vi "Toolkit - Cluster Constant.vi"() -> ()   [LabVIEW 2017]
doc: "Alphabetizes a cluster constant using VI scripting and the ACE toolkit VIs"
uses:
  <vilib>/Utility/traverseref.llb/TRef TravTarget.ctl
  Toolkit/Toolkit.lvlib
  <vilib>/Utility/traverseref.llb/VI Scripting - Traverse.lvlib
panel:
  out "Change?":bool
  # "Overview: Demonstrates alphabetizing a cluster constant using VI scripting the ACE toolkit\nInstructions:\n1. Run this VI"
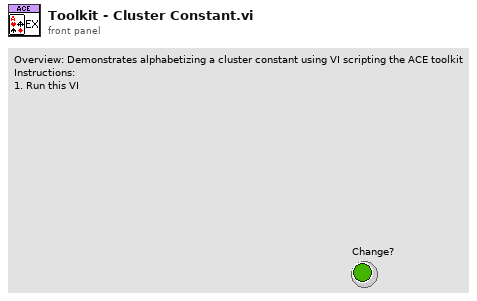
[diagram p1: front panel]
types:
  T1 = enum32{"Invalid", "Standard", "Closed", "Hidden", "Minimized", "Maximized"}
  T2 = typedef "TRef TravTarget.ctl" = enum16{"FP", "BD", "Other"}
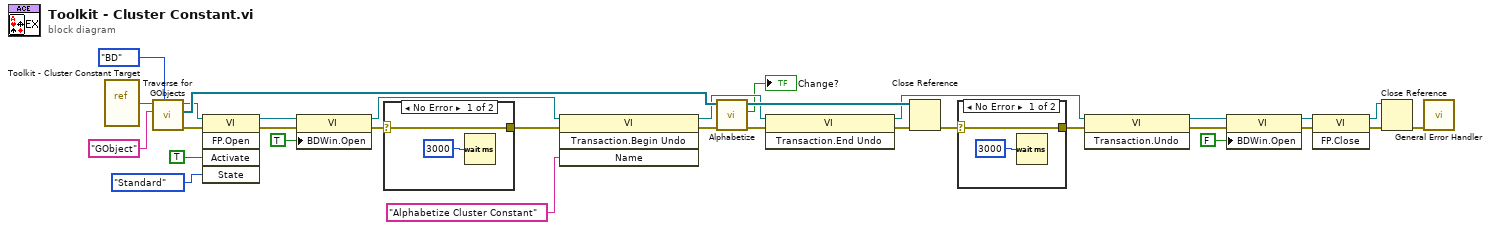
[diagram p0: block diagram]
diagram:
  n1 = vi-ref "Toolkit - Cluster Constant Target.vi"() -> (w17:refnum<vi>)
  n2 = call <vilib>:"Traverse for GObjects.vi"("Traverse Target"=TRef_TravTarget."BD", "Class Name"="GObject", "VI Refnum"=w17) -> ("error out"=w25:errorcluster, "References"=w30:refnum<vi>[], "dup VI Refnum"=w24:refnum<vi>)  [unwired: 5 in, 1 out]
  n3 = invoke class="VI" method="FP.Open"(reference=w24, error in=w25, "Activate"=TRUE ("Activate?"), "State"=T1."Standard") -> (reference out=w23:refnum<vi>, error out=w22:errorcluster)  [unwired: 1 in, 3 out]
  n4 = property class="VI"(reference=w23, error in=w22, "BDWin.Open"=TRUE ("Block Diagram Window:Open")) -> (reference out=w14:refnum<vi>, error out=w20:errorcluster)
  n5 = case shown="No Error" w20 {
    selector: w20 -> [w34 w35]
    tunnel: [w34 w35] -> w16
    frame No Error {
      n6 = Wait (ms)(milliseconds to wait=u32 3000) -> ()  [unwired: 1 out]
    }
    frame Error {
    }
  }
  n7 = invoke class="VI" method="Transaction.Begin Undo"(reference=w14, error in=w16, "Name"="Alphabetize Cluster Constant") -> (reference out=w11:refnum<vi>, error out=w15:errorcluster)  [unwired: 1 in, 2 out]
  n8 = call "Alphabetize.vi"("Error In"=w15, "Clusters In"=w30) -> ("Error Out"=w12:errorcluster, "Change?"=→"Change?":bool, "Clusters Out"=w28:refnum<vi>[])  [unwired: 7 in]
  n9 = invoke class="VI" method="Transaction.End Undo"(reference=w11, error in=w12) -> (reference out=w9:refnum<vi>, error out=w10:errorcluster)  [unwired: 1 in, 1 out]
  n10 = Close Reference(reference=w28, error in (no error)=w10) -> (error out=w19:errorcluster)
  n11 = case shown="No Error" w19 {
    selector: w19 -> [w37 w38]
    tunnel: [w37 w38] -> w18
    frame No Error {
      n12 = Wait (ms)(milliseconds to wait=u32 3000) -> ()  [unwired: 1 out]
    }
    frame Error {
    }
  }
  n13 = invoke class="VI" method="Transaction.Undo"(reference=w9, error in=w18) -> (reference out=w8:refnum<vi>, error out=w7:errorcluster)  [unwired: 1 in, 1 out]
  n14 = property class="VI"(reference=w8, error in=w7, "BDWin.Open"=FALSE ("Block Diagram Window:Open")) -> (reference out=w5:refnum<vi>, error out=w2:errorcluster)
  n15 = invoke class="VI" method="FP.Close"(reference=w5, error in=w2) -> (reference out=w4:refnum<vi>, error out=w3:errorcluster)  [unwired: 1 in, 1 out]
  n16 = Close Reference(reference=w4, error in (no error)=w3) -> (error out=w29:errorcluster)
  n17 = call <vilib>:"General Error Handler.vi"("error in (no error)"=w29) -> ()  [unwired: 10 in, 5 out]
